vi "NetworkSettingsDialog.vi"(8 "error in (no error)":errorcluster, 11 "Network In":T1={"invert_send"=TRUE, "Number of datagrams to read"=5000, "max bytes/read"=2500, "Timeout"=4000, "host"="192.168.1.18", "Port Receive"=5678} {"Number of datagrams to read" format="%0d"}) -> (0 "error out":errorcluster, 2 "UI Refresh Needed?":bool, 3 "Network Out":T1={"invert_send"=TRUE, "Number of datagrams to read"=5000, "max bytes/read"=2500, "Timeout"=4000, "host"="192.168.1.18", "Port Receive"=5678} {"Number of datagrams to read" format="%0d"})   [LabVIEW 2014]
uses:
  controls/Network.ctl
panel:
  out "found":bool
  in  "Ping":bool
  in  "Timeout":dbl=4000.0
  in  "port receive address":dbl=5678.0
  in  "maximum bytes":dbl=2500.0
  in  "invert":bool=TRUE
  in  "Datagram to read":dbl=5000.0
  in  "host":string="192.168.1.18"
  in  "Cancel Button":bool
  in  "OK Button":bool
  # "Network settings"
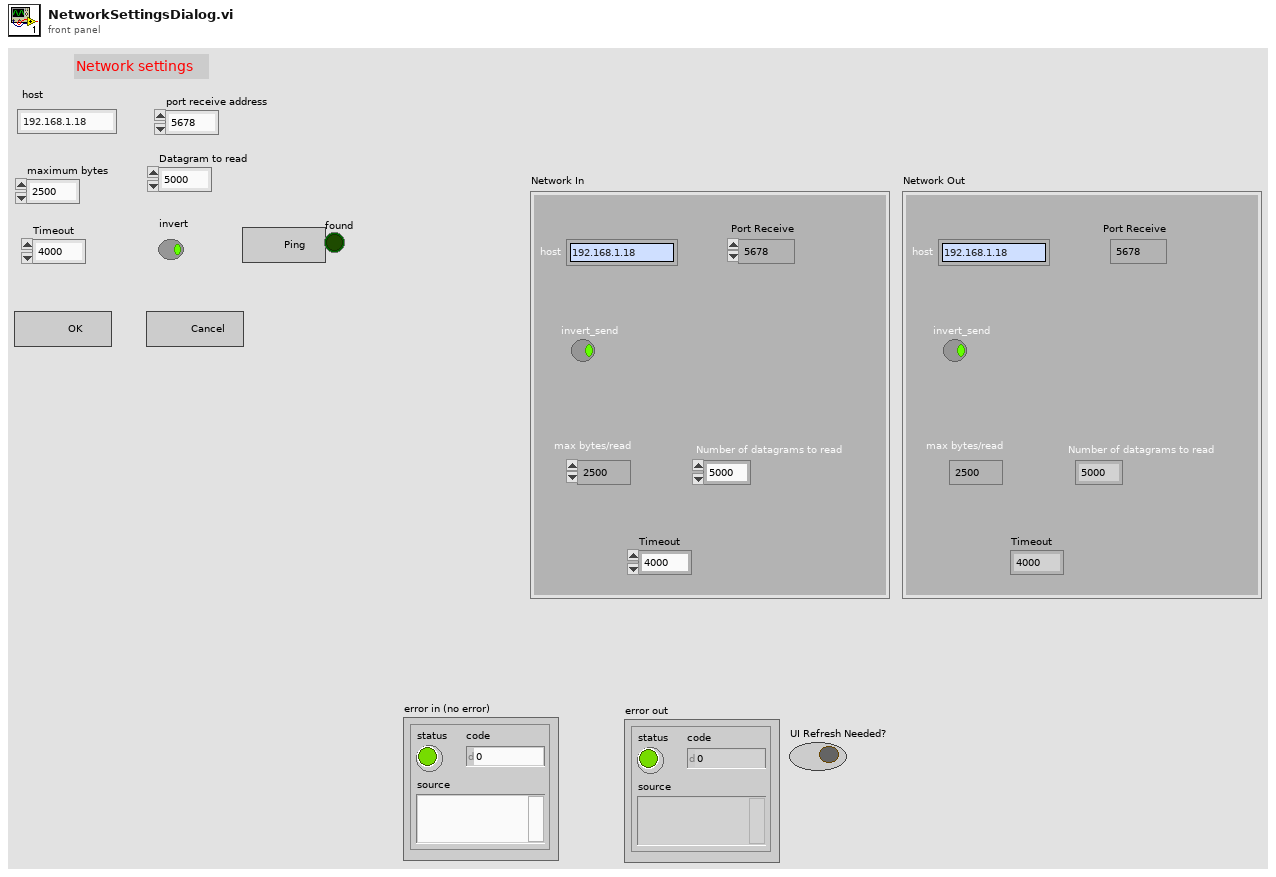
[diagram p1: front panel]
types:
  T1 = typedef "Network.ctl" = cluster{"invert_send":bool, "Number of datagrams to read":u32, "max bytes/read":i32, "Timeout":i32, "host":string, "Port Receive":u16}
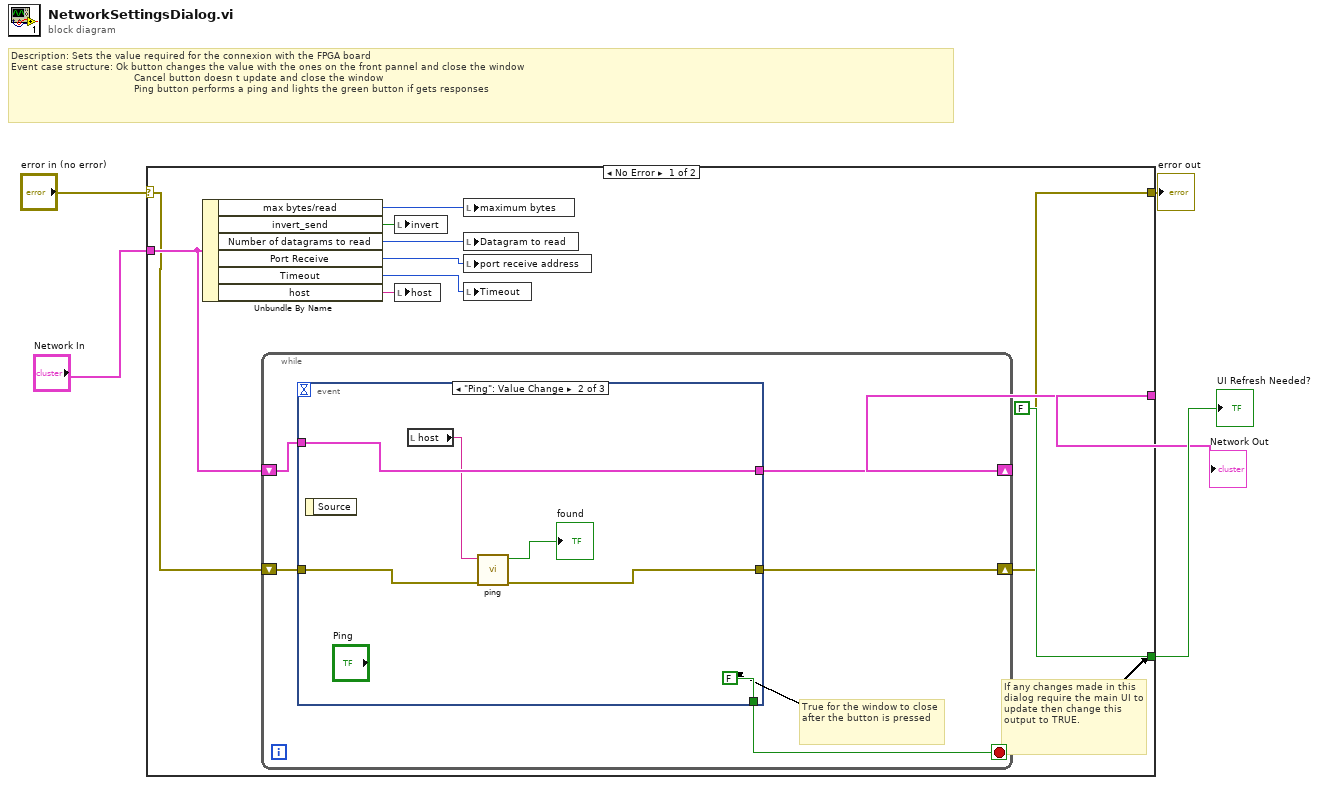
[diagram p0: block diagram]
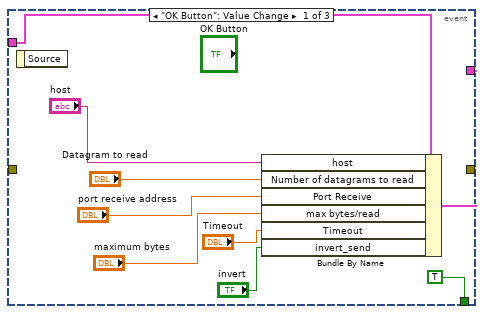
[diagram p2: hidden frame]
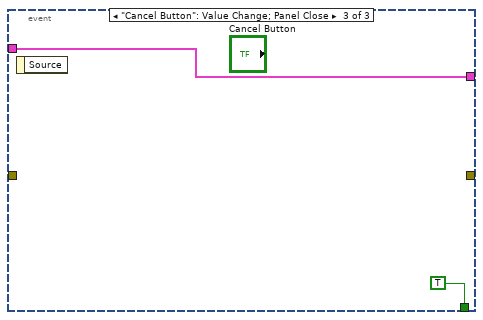
[diagram p3: hidden frame]
diagram:
  # "Description: Sets the value required for the connexion with the FPGA board\nEvent case structure: Ok button changes the value with the ones on the front pannel and close the window\n                                         Cancel button doesn t update and close the window\n                                         Ping button performs a ping and lights the green button if gets responses"
  n1 = case shown="No Error" "error in (no error)" {
    selector: "error in (no error)" -> [w7 w40]
    tunnel: [w6 w40] -> w4
    tunnel: "Network In" -> [w14 w39]
    tunnel: [w16 w39] -> w1
    tunnel: [FALSE ("UI Refresh Needed?") _] -> w3
    frame No Error {
      # "If any changes made in this dialog require the main UI to update then change this output to TRUE."
      n2 = Unbundle By Name(w14) -> ("max bytes/read"=w12:i32, "invert_send"=w13:bool, "Number of datagrams to read"=w10:u32, "Port Receive"=w11:u16, "Timeout"=w9:i32, "host"=w8:string)
      n3 = while {
        shift-right: [w21] -> w16
        shift-left: w14 -> [w20]
        shift-right: [w18] -> w6
        shift-left: w7 -> [w19]
        stop <- w17 stop-if-true
        # "True for the window to close after the button is pressed"
        n4 = event shown="[1] \"Ping\": Value Change" {
          selector: _ -> [_ _ _]
          dyn-events: _ -> [_ _ _]
          timeout: _ -> [_ _ _]
          tunnel: [w24 w33 w38] -> w21
          tunnel: w20 -> [w30 w33 w38]
          tunnel: w19 -> [_ w36 _]
          tunnel: [_ w35 _] -> w18
          tunnel: [TRUE FALSE TRUE] -> w17
          event "OK Button": Value Change {
            n5 = event-data() -> ()  [unwired: 1 in, 1 out]
            n6 = Bundle By Name(cluster=w30, "host"="host", "Number of datagrams to read"="Datagram to read", "Port Receive"="port receive address", "max bytes/read"="maximum bytes", "Timeout"="Timeout", "invert_send"="invert") -> (w24:T1)
          }
          event "Ping": Value Change {
            n7 = event-data() -> ()  [unwired: 1 in, 1 out]
            n8 = local read "host"() -> (w31:string)
            n9 = call "ping.vi"("error in"=w36, "host"=w31) -> ("error out"=w35:errorcluster, "found"=→"found":bool)  [unwired: 8 in]
          }
          event "Cancel Button": Value Change; Panel Close {
            n10 = event-data() -> ()  [unwired: 1 in, 1 out]
          }
        }
      }
      n11 = local write "invert"(w13) -> ()
      n12 = local write "host"(w8) -> ()
      n13 = local write "maximum bytes"(w12) -> ()
      n14 = local write "Datagram to read"(w10) -> ()
      n15 = local write "port receive address"(w11) -> ()
      n16 = local write "Timeout"(w9) -> ()
    }
    frame Error {
    }
  }
  "UI Refresh Needed?" <- w3
  "error out" <- w4
  "Network Out" <- w1
